vi "DataFile_Format.vi"() -> ()   [LabVIEW 2020]
uses:
  DataCluster.ctl
  <vilib>/userdefined/High Color/IMAQdx.ctl
  <vilib>/vision/Image Controls.llb/IMAQ Image.ctl
panel:
  out "Array":string[][](array[string])
  in  "DataCluster":T1 {"System"."Setup"."TargetTemp" min=-30.0 max=30.0 step=0.5 format="%#_g °C"; "System"."Setup"."TempGrad" min=-100.0 max=100.0 step=0.1 format="%#_g °C/min"}
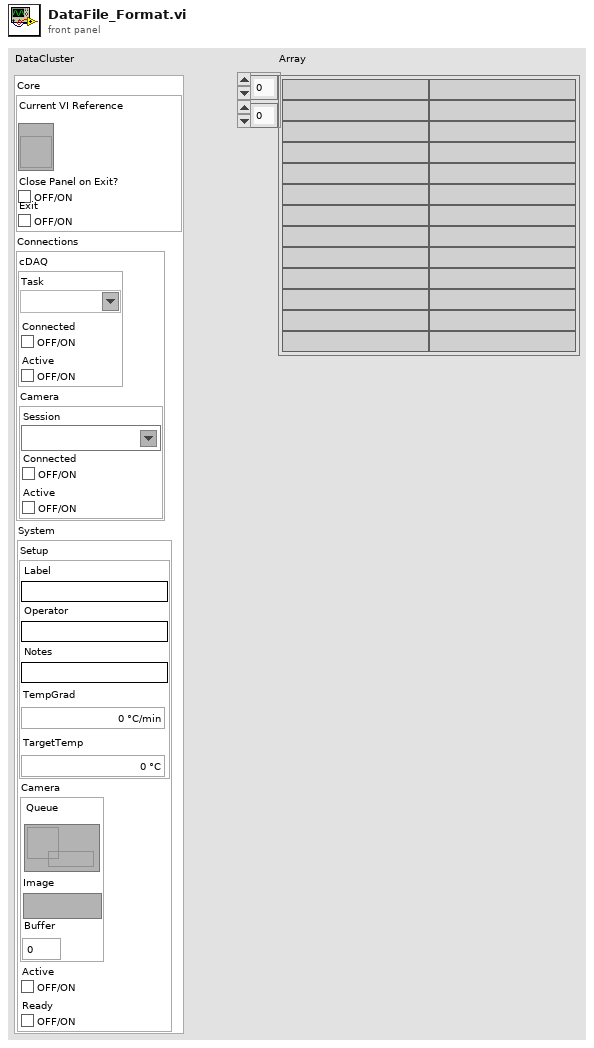
[diagram p1: front panel]
types:
  T1 = typedef "DataCluster.ctl" = cluster{"Core":cluster{"Current VI Reference":refnum<vi>, "Close Panel on Exit?":bool, "Exit":bool}, "Connections":cluster{"cDAQ":cluster{"Task":refnum<k21>, "Connected":bool, "Active":bool}, "Camera":cluster{"Session":T2, "Connected":bool, "Active":bool}}, "System":cluster{"Setup":cluster{"Label":string, "Operator":string, "Notes":string, "TempGrad":dbl, "TargetTemp":dbl}, "Camera":cluster{"Queue":refnum<queue>, "Image":T3, "Buffer":dbl}, "Active":bool, "Ready":bool}}
  T2 = typedef "IMAQdx.ctl" = refnum<k21>
  T3 = typedef "IMAQ Image.ctl" = refnum<image>
  T4 = cluster{"Label":string, "Operator":string, "Notes":string, "TempGrad":dbl, "TargetTemp":dbl}
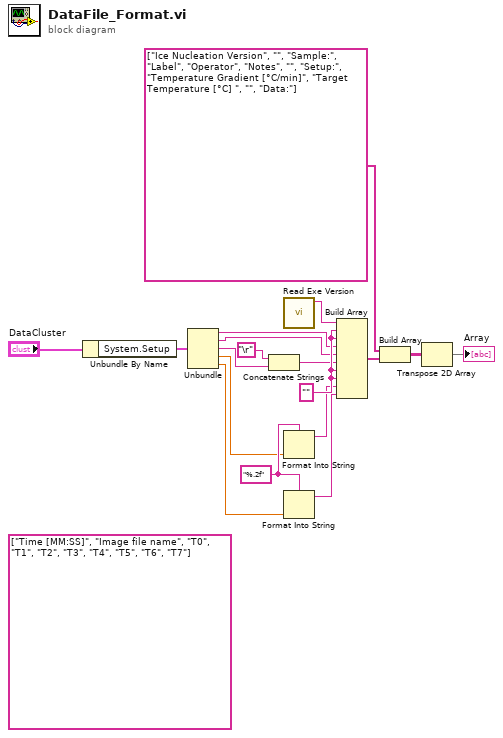
[diagram p0: block diagram]
diagram:
  (unwired) string[] ["Time [MM:SS]", "Image file name", "T0", "T1", "T2", "T3", "T4", "T5", "T6", "T7"]
  w13 = "%.2f" ("format string")
  w17 = "" ("element")
  n1 = Unbundle By Name("DataCluster") -> ("System.Setup"=w6:T4)
  n2 = Unbundle(w6) -> ("Label"=w8:string, "Operator"=w1:string, "Notes"=w3:string, "TempGrad"=w9:dbl, "TargetTemp"=w11:dbl)
  n3 = Concatenate Strings("\r", w3) -> (w2:string)
  n4 = call "Read Exe Version.vi"() -> ("FileVersion"=w7:string)  [unwired: 10 in, 1 out]
  n5 = Format Into String(format string=w13, w9) -> (resulting string=w10:string)  [unwired: 2 in, 1 out]
  n6 = Format Into String(format string=w13, w11) -> (resulting string=w12:string)  [unwired: 2 in, 1 out]
  n7 = Build Array(w7, w17, w17, w8, w1, w2, w17, w17, w10, w12) -> (w14:string[])
  n8 = Build Array(string[] ["Ice Nucleation Version", "", "Sample:", "Label", "Operator", "Notes", "", "Setup:", "Temperature Gradient [°C/min]", "Target Temperature [°C] ", "", "Data:"], w14) -> (w16:string[][])
  n9 = Transpose 2D Array(2D array=w16) -> (transposed array=→"Array":string[][])
